vi "Read.vi"(8 "error in (no error)":errorcluster) -> (0 "error out":errorcluster, 2 "Character":i32)   [LabVIEW 2017, in "MGI-Console.lvlib" / "Console.lvclass"]
doc: "The next character from the input stream, or negative one (-1) if there are currently no more characters to be read.\n----\nCopyright: MGI 2018\nAuthor: Derek Trepanier"
uses:
  Console.lvclass
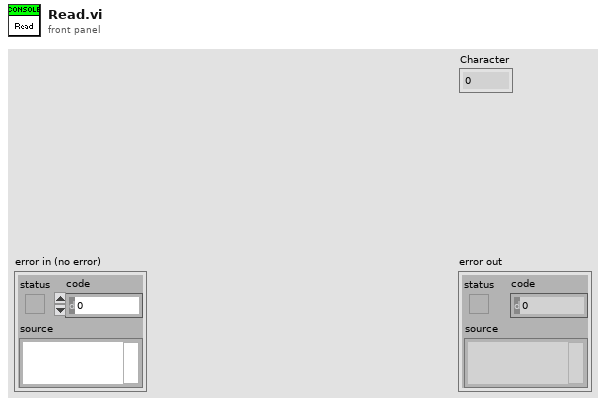
[diagram p1: front panel]
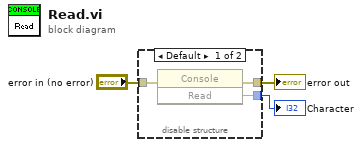
[diagram p0: block diagram]
diagram:
  n1 = disable-structure shown="Default" {
    disable-tunnel: "error in (no error)" -> [w6 w7]
    disable-tunnel: [w5 w7] -> w2
    disable-tunnel: [w4 _] -> w1
    frame condition #0 {
      n2 = invoke class="Console" method="Read"(error in=w6) -> (error out=w5:errorcluster, "Read"=w4:i32)  [unwired: 2 in, 1 out]
    }
    frame condition #1 (active) {
    }
  }
  "error out" <- w2
  "Character" <- w1
